vi "Bezier Spline.vi"(6 "positions":cluster{dbl[]}[](array[cluster]), 8 "ending orientation (deg)":sgl=nan, 9 "starting orientation (deg)":sgl=nan, 10 "percision":sgl=0.01, 11 "waypts":cluster{"x":sgl, "y":sgl}[](array[cluster])) -> (0 "cubic spline ctrl pts":cluster{sgl, sgl}[][](array[cluster]), 1 "Tangents":cluster{sgl, sgl}[](array[cluster]), 2 "ctrl pts":cluster{sgl, sgl}[][](array[cluster]), 3 "bezier spline":cluster{"curve ":T1}[](array[cluster]), 4 "position out":sgl[][](array[numeric]))   [LabVIEW 2025]
uses:
  Types/Bezier Curve.ctl
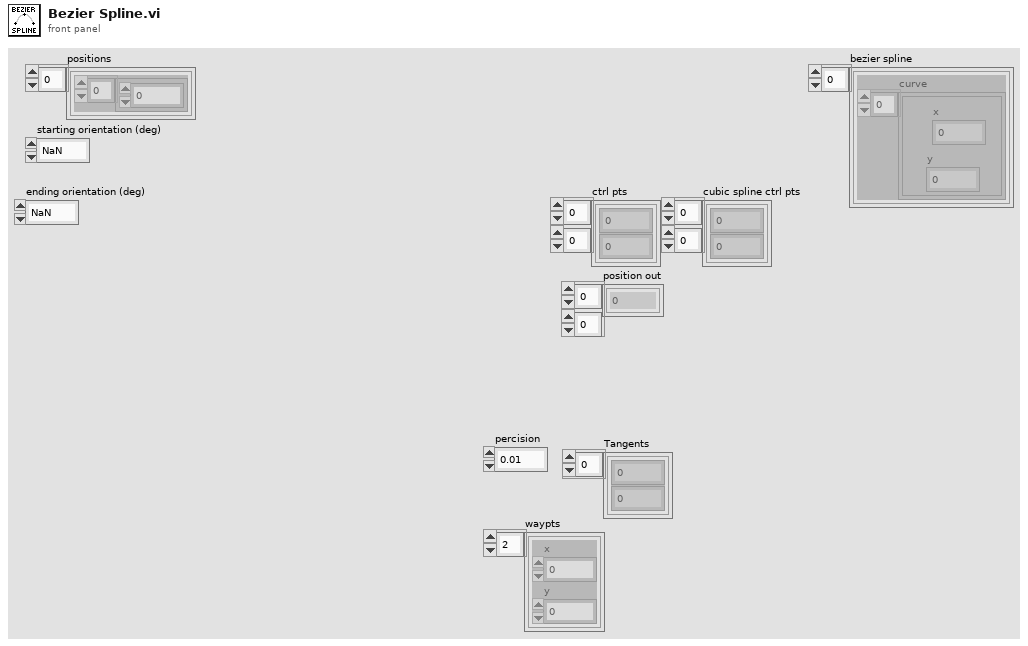
[diagram p1: front panel]
types:
  T1 = typedef "Bezier Curve.ctl" = cluster{"x":sgl, "y":sgl}[]
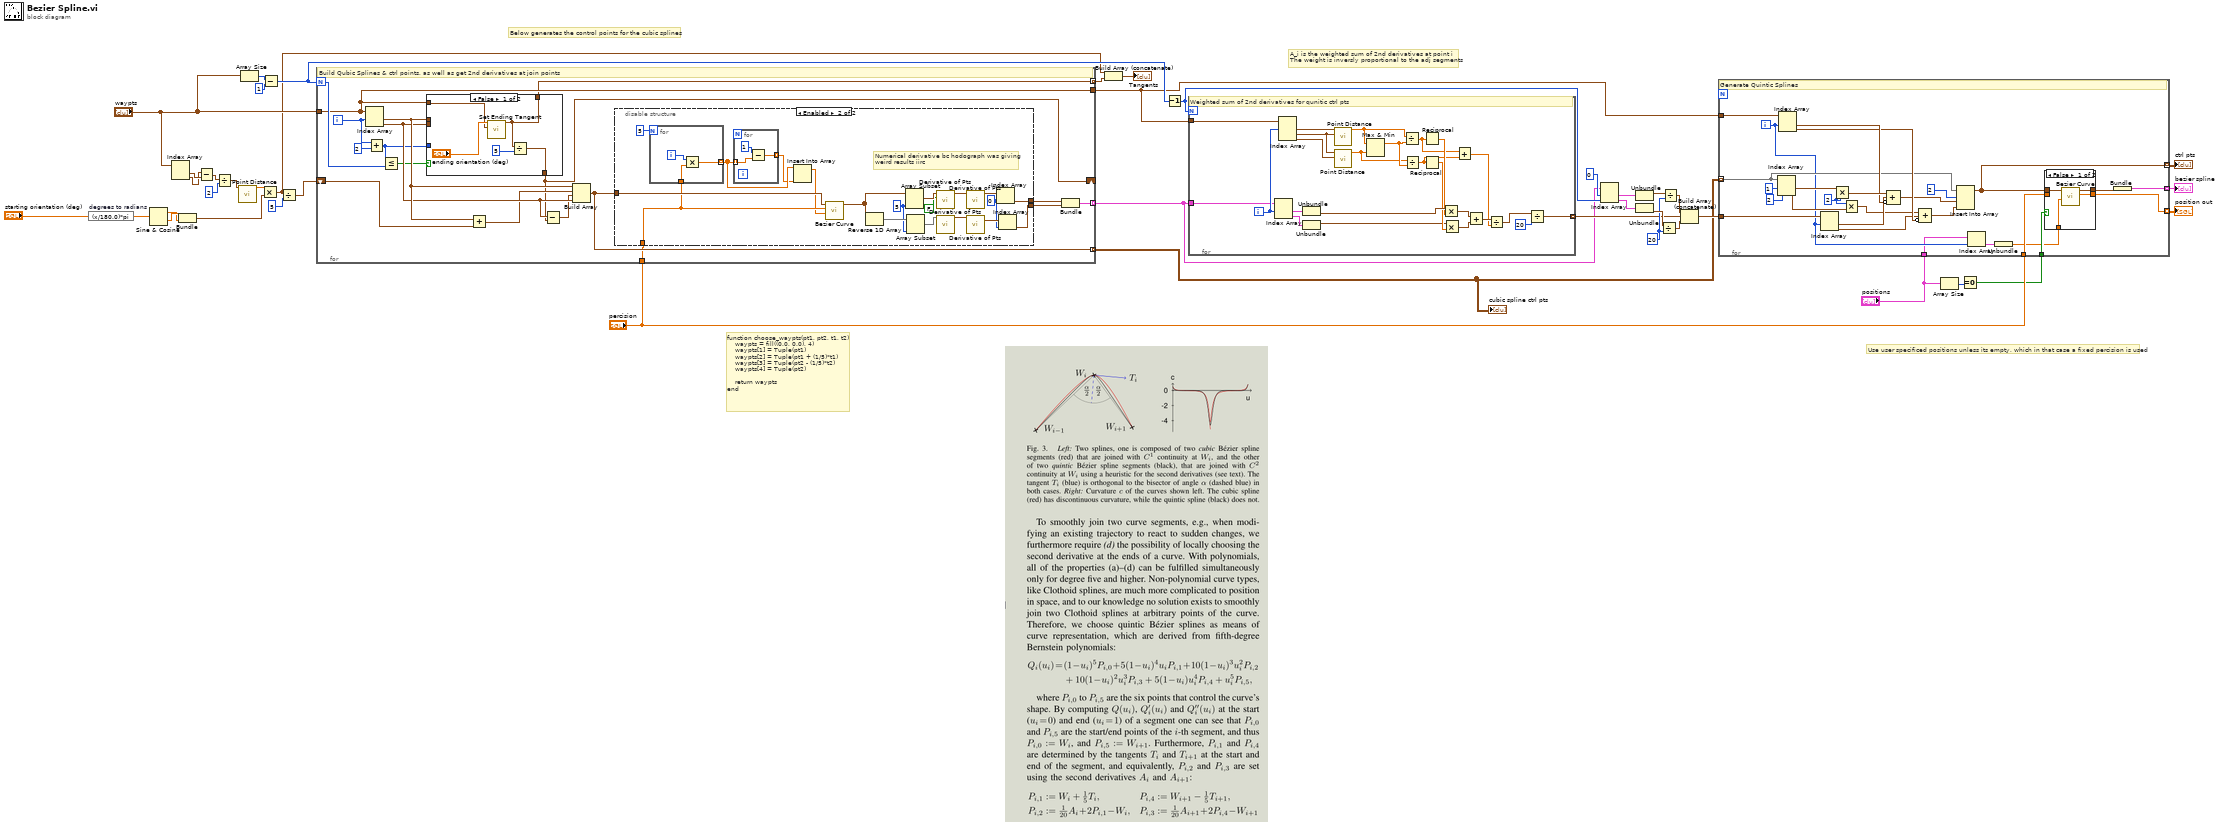
[diagram p0: block diagram]
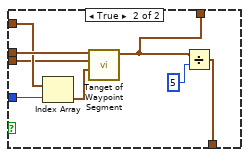
[diagram p2: hidden frame]
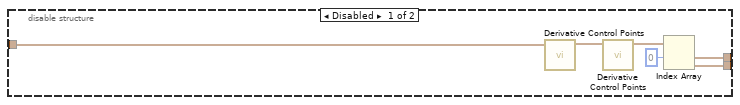
[diagram p3: hidden frame]
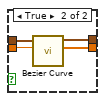
[diagram p4: hidden frame]
diagram:
  w24 = 20
  # "function choose_waypts(pt1, pt2, t1, t2)\n    waypts = fill((0.0, 0.0), 4)\n    waypts[1] = Tuple(pt1)\n    waypts[2] = Tuple(pt1 + (1/5)*t1)\n    waypts[3] = Tuple(pt2 - (1/5)*t2)\n    waypts[4] = Tuple(pt2)\n\n    return waypts\nend"
  # "Use user specificed positions unless its empty, which in that case a fixed percision is used"
  # "Below generates the control points for the cubic splines"
  # "A_i is the weighted sum of 2nd derivatives at point i\nThe weight is inversly proportional to the adj segments"
  n1 = expression code="(x/180.0)*pi" "degrees to radians"("starting orientation (deg)") -> (w14:sgl)
  n2 = Sine & Cosine(0:w14) -> (1:w12:sgl, 2:w13:sgl)
  n3 = Index Array(array="waypts") -> (element #1=w39:cluster{"x":sgl, "y":sgl}, element #2=w38:cluster{"x":sgl, "y":sgl})  [unwired: 2 in]
  n4 = Bundle(w13, w12) -> (w35:cluster{sgl, sgl})  [unwired: 1 in]
  n5 = Subtract(x=w38, y=w39) -> (x-y=w37:cluster{"x":sgl, "y":sgl})
  n6 = Divide(x=w37, y=u16 2) -> (x/y=w18:cluster{"x":sgl, "y":sgl})
  n7 = call "Point Distance.vi"("point a"=w18) -> ("dist"=w19:sgl)  [unwired: 10 in]
  n8 = Array Size(array="waypts") -> (size(s)=w41:i32)
  n9 = Multiply(x=w19, y=w35) -> (x*y=w8:cluster{sgl, sgl})
  n10 = Subtract(x=w41, y=1) -> (x-y=w33:i32)
  n11 = Divide(x=w8, y=u16 5) -> (x/y=w16:cluster{sgl, sgl})
  n12 = for {
    N: w33 -> [w48]
    tunnel: "waypts" -> [w47]
    shift-right: [w46] -> _
    shift-left: w16 -> [w50]
    tunnel: [w45] -> w5 mode=indexing
    tunnel: [w53] -> w10 mode=indexing
    tunnel: [w47] -> w11
    tunnel: "percision" -> [w44]
    tunnel: [w43] -> w17 mode=indexing
    i -> [w52]
    # "Build Qubic Splines & ctrl points, as well as get 2nd derivatives at join points"
    n13 = Index Array(array=w47, index #1=w52) -> (element #1=w59:cluster{"x":sgl, "y":sgl}, element #2=w58:cluster{"x":sgl, "y":sgl})  [unwired: 1 in]
    n14 = Add(x=w52, y=2) -> (x+y=w49:i32)
    n15 = Less Or Equal?(x=w49, y=w48) -> (x <= y?=w42:bool)
    n16 = case shown="False" w42 {
      tunnel: w59 -> [_ w72]
      tunnel: w58 -> [_ w66]
      tunnel: [w61 w70] -> w46
      tunnel: w49 -> [_ w69]
      tunnel: w47 -> [w62 w68]
      tunnel: [w60 w65] -> w43
      frame False {
        n17 = call "Set Ending Tangent.vi"("waypts"=w62, "ending orientation"="ending orientation (deg)") -> ("ending tangent"=w60:cluster{sgl, sgl})  [unwired: 9 in]
        n18 = Divide(x=w60, y=u16 5) -> (x/y=w61:cluster{sgl, sgl})
      }
      frame True {
        n19 = Index Array(array=w68, index=w69) -> (element=w67:cluster{"x":sgl, "y":sgl})
        n20 = call "Tanget of Waypoint Segment.vi"("point c"=w67, "point b"=w66, "point a"=w72) -> ("T_i"=w65:cluster{sgl, sgl})  [unwired: 8 in]
        n21 = Divide(x=w65, y=u16 5) -> (x/y=w70:cluster{sgl, sgl})
      }
    }
    n22 = Add(x=w59, y=w50) -> (x+y=w57:cluster{sgl, sgl})
    n23 = Subtract(x=w58, y=w46) -> (x-y=w56:cluster{sgl, sgl})
    n24 = Build Array(w59, w57, w56, w58) -> (w45:cluster{"x":sgl, "y":sgl}[])
    n25 = disable-structure shown="Enabled" {
      disable-tunnel: w45 -> [w77 w85]
      disable-tunnel: [w74 w88] -> w55
      disable-tunnel: [w73 w87] -> w54
      disable-tunnel: w44 -> [_ w83]
      frame Disabled {
        n26 = call "Derivative Control Points.vi"("ctrl points"=w77) -> ("d ctrl pts"=w78:cluster{dbl, dbl}[])  [unwired: 10 in]
        n27 = call "Derivative Control Points.vi"("ctrl points"=w78) -> ("d ctrl pts"=w76:cluster{dbl, dbl}[])  [unwired: 10 in]
        n28 = Index Array(array=w76, index #1=0 ("index")) -> (element #1=w74:cluster{dbl, dbl}, element #2=w73:cluster{dbl, dbl})  [unwired: 1 in]
      }
      frame Enabled {
        w90 = 0 ("index")
        w89 = 5 ("length")
        # "Numerical derivative bc hodograph was giving\nweird results iirc"
        n29 = for {
          N: 5 -> [_]
          tunnel: w83 -> [w102]
          tunnel: [w101] -> w80 mode=indexing
          i -> [w103]
          n30 = Multiply(x=w103, y=w102) -> (x*y=w101:sgl)
        }
        n31 = for {
          tunnel: w80 -> [w100] mode=indexing
          tunnel: [w98] -> w79 mode=indexing
          n32 = Subtract(x=1 ("length"), y=w100) -> (x-y=w98:sgl)
        }
        n33 = Insert Into Array(array=w80, new element=w79) -> (w82:sgl[])  [unwired: 1 in]
        n34 = call "Bezier Curve.vi"("position"=w82, "percision"=w83, "ctrl points"=w85) -> ("curve"=w81:T1)  [unwired: 7 in, 1 out]
        n35 = Reverse 1D Array(array=w81) -> (reversed array=w97:T1)
        n36 = Array Subset(array=w81, length=w89) -> (w96:T1)  [unwired: 1 in]
        n37 = Array Subset(array=w97, length=w89) -> (w94:T1)  [unwired: 1 in]
        n38 = call "Derivative of Pts.vi"("pts"=w94) -> ("pts out"=w93:cluster{sgl, sgl}[])  [unwired: 10 in]
        n39 = call "Derivative of Pts.vi"("fix first pt?"=FALSE, "pts"=w96) -> ("pts out"=w95:cluster{sgl, sgl}[])  [unwired: 9 in]
        n40 = call "Derivative of Pts.vi"("pts"=w95) -> ("pts out"=w92:cluster{sgl, sgl}[])  [unwired: 10 in]
        n41 = call "Derivative of Pts.vi"("pts"=w93) -> ("pts out"=w91:cluster{sgl, sgl}[])  [unwired: 10 in]
        n42 = Index Array(array=w92, index=w90) -> (element=w88:cluster{sgl, sgl})
        n43 = Index Array(array=w91, index=w90) -> (element=w87:cluster{sgl, sgl})
      }
    }
    n44 = Bundle(w55, w54) -> (w53:cluster{cluster{sgl, sgl}, cluster{sgl, sgl}})  [unwired: 1 in]
  }
  "cubic spline ctrl pts" <- w5
  n45 = Build Array (concatenate)(w8, w17) -> (→"Tangents":cluster{sgl, sgl}[])
  n46 = Decrement(x=w33) -> (x-1=w28:i32)
  n47 = for {
    N: w28 -> [_]
    tunnel: w10 -> [w118]
    tunnel: w11 -> [w117]
    tunnel: [w107] -> w20 mode=indexing
    i -> [w127]
    # "Weighted sum of 2nd derivatives for qunitic ctrl pts"
    n48 = Index Array(array=w118, index #1=w127) -> (element #1=w126:cluster{cluster{sgl, sgl}, cluster{sgl, sgl}}, element #2=w125:cluster{cluster{sgl, sgl}, cluster{sgl, sgl}})  [unwired: 1 in]
    n49 = Index Array(array=w117, index #1=w127) -> (element #1=w124:cluster{"x":sgl, "y":sgl}, element #2=w123:cluster{"x":sgl, "y":sgl}, element #3=w122:cluster{"x":sgl, "y":sgl})  [unwired: 2 in]
    n50 = Unbundle(w126) -> (w115:cluster{sgl, sgl})  [unwired: 1 out]
    n51 = Unbundle(w125) -> (w112:cluster{sgl, sgl})  [unwired: 1 out]
    n52 = call "Point Distance.vi"("point b"=w123, "point a"=w124) -> ("dist"=w121:sgl)  [unwired: 9 in]
    n53 = call "Point Distance.vi"("point b"=w122, "point a"=w123) -> ("dist"=w119:sgl)  [unwired: 9 in]
    n54 = Max & Min(x=w121, y=w119) -> (max(x,y)=w120:sgl)  [unwired: 1 out]
    n55 = Divide(x=w121, y=w120) -> (x/y=w106:sgl)
    n56 = Divide(x=w119, y=w120) -> (x/y=w105:sgl)
    n57 = Reciprocal(x=w106) -> (1/x=w114:sgl)
    n58 = Reciprocal(x=w105) -> (1/x=w113:sgl)
    n59 = Multiply(x=w115, y=w114) -> (x*y=w111:cluster{sgl, sgl})
    n60 = Multiply(x=w112, y=w113) -> (x*y=w110:cluster{sgl, sgl})
    n61 = Add(x=w106, y=w105) -> (x+y=w104:sgl)
    n62 = Add(x=w111, y=w110) -> (x+y=w109:cluster{sgl, sgl})
    n63 = Divide(x=w109, y=w104) -> (x/y=w108:cluster{sgl, sgl})
    n64 = Divide(x=w108, y=20) -> (x/y=w107:cluster{sgl, sgl})
  }
  n65 = Index Array(array=w10, index #1=0 ("index"), index #2=w28) -> (element #1=w32:cluster{cluster{sgl, sgl}, cluster{sgl, sgl}}, element #2=w30:cluster{cluster{sgl, sgl}, cluster{sgl, sgl}})
  n66 = Unbundle(w32) -> (w25:cluster{sgl, sgl})  [unwired: 1 out]
  n67 = Unbundle(w30) -> (w27:cluster{sgl, sgl})  [unwired: 1 out]
  n68 = Divide(x=w27, y=w24) -> (x/y=w26:cluster{sgl, sgl})
  n69 = Divide(x=w25, y=w24) -> (x/y=w23:cluster{sgl, sgl})
  n70 = Build Array (concatenate)(w23, w20, w26) -> (w31:cluster{sgl, sgl}[])
  n71 = Array Size(array="positions") -> (size(s)=w6:i32)
  n72 = Equal To 0?(x=w6) -> (x = 0?=w3:bool)
  n73 = for {
    tunnel: w31 -> [w151]
    tunnel: w5 -> [w134] mode=indexing
    tunnel: w11 -> [w152]
    tunnel: "percision" -> [w138]
    tunnel: [w137] -> w22 mode=indexing
    tunnel: [w136] -> w7 mode=indexing
    tunnel: w3 -> [w135]
    tunnel: "positions" -> [w132]
    tunnel: [w128] -> w2 mode=indexing
    i -> [w133]
    w148 = u16 2
    # "Generate Quintic Splines"
    n74 = Index Array(array=w134, index #1=1 ("index"), index #2=2 ("index")) -> (element #1=w150:cluster{"x":sgl, "y":sgl}, element #2=w149:cluster{"x":sgl, "y":sgl})
    n75 = Index Array(array=w152, index #1=w133) -> (element #1=w145:cluster{"x":sgl, "y":sgl}, element #2=w144:cluster{"x":sgl, "y":sgl})  [unwired: 1 in]
    n76 = Index Array(array=w151, index #1=w133) -> (element #1=w146:cluster{sgl, sgl}, element #2=w142:cluster{sgl, sgl})  [unwired: 1 in]
    n77 = Multiply(x=w150, y=w148) -> (x*y=w147:cluster{"x":sgl, "y":sgl})
    n78 = Multiply(x=w148, y=w149) -> (x*y=w143:cluster{"x":sgl, "y":sgl})
    n79 = Compound Arithmetic op=ADD(w147, w146, invert w145) -> (w141:cluster{sgl, sgl})
    n80 = Compound Arithmetic op=ADD(w143, w142, invert w144) -> (w140:cluster{sgl, sgl})
    n81 = Insert Into Array(array=w134, index=2, new element #1=w141, new element #2=w140) -> (w137:cluster{"x":sgl, "y":sgl}[])
    n82 = Index Array(array=w132, index=w133) -> (element=w131:cluster{dbl[]})
    n83 = Unbundle(w131) -> (w130:dbl[])
    n84 = case shown="False" w135 {
      tunnel: w138 -> [_ w162]
      tunnel: [w157 w161] -> w129
      tunnel: w137 -> [w158 w160]
      tunnel: [w156 w159] -> w136
      tunnel: w130 -> [w155 _]
      frame False {
        n85 = call "Bezier Curve.vi"("position"=w155, "ctrl points"=w158) -> ("position out"=w156:sgl[], "curve"=w157:T1)  [unwired: 8 in]
      }
      frame True {
        n86 = call "Bezier Curve.vi"("percision"=w162, "ctrl points"=w160) -> ("position out"=w159:sgl[], "curve"=w161:T1)  [unwired: 8 in]
      }
    }
    n87 = Bundle("curve"=w129) -> (w128:cluster{"curve ":T1})  [unwired: 1 in]
  }
  "ctrl pts" <- w22
  "position out" <- w7
  "bezier spline" <- w2
